vi "Dvr Caller.vi"(6 "Sub Panel":refnum<vi>, 8 "Error In":errorcluster, 11 "Data Value Reference In":refnum<data-value>) -> (0 "Error Out":errorcluster, 3 "Data Value Reference Out":refnum<data-value>)   [LabVIEW 2021, in "Calculator.lvlib" / "NumericOperation.lvclass"]
doc: "This VI acts a wrapper VI which gets the subpanel reference as input and calls an overriding method Caller corresponding to the Data Value Reference."
uses:
  NumericOperation.lvclass
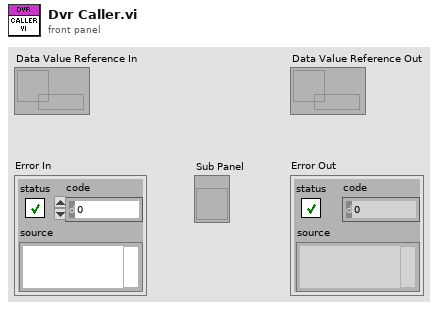
[diagram p1: front panel]
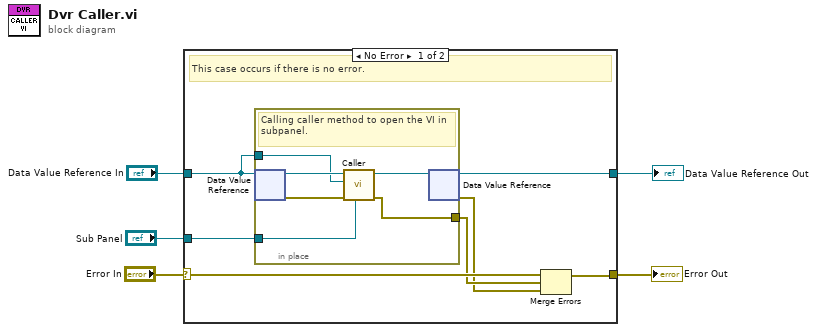
[diagram p0: block diagram]
diagram:
  n1 = case shown="No Error" "Error In" {
    selector: "Error In" -> [w10 w20]
    tunnel: [w7 w20] -> w4
    tunnel: "Data Value Reference In" -> [w6 w19]
    tunnel: [w12 w19] -> w2
    tunnel: "Sub Panel" -> [w11 _]
    frame No Error {
      # "This case occurs if there is no error."
      n2 = in-place {
        in-place-border: w11 -> [w16]
        in-place-border: [w14] -> w9
        in-place-border: w6 -> [w13]
        # "Calling caller method to open the VI in subpanel."
        n3 = in-place-dvr #1(w6) -> (w18:refnum<class "NumericOperation.lvclass">, w15:errorcluster)
        n4 = call-dynamic "Caller.vi"("Sub Panel"=w16, "Error In"=w15, "Data Value Reference In"=w13, "NumericOperation in"=w18) -> ("Error Out"=w14:errorcluster, "NumericOperation out"=w17:refnum<class "NumericOperation.lvclass">)  [unwired: 6 in]
        n5 = in-place-dvr #1(w17) -> (w12:refnum<data-value>, w8:errorcluster)
      }
      n6 = Merge Errors(w10, w9, w8) -> (w7:errorcluster)
    }
    frame Error {
      # "This case occurs if there is any error."
    }
  }
  "Error Out" <- w4
  "Data Value Reference Out" <- w2
